vi "Inventory-Add#toIventory.vi"(7 "Quanity to Add/Subtract":i32, 8 "error in (no error)":errorcluster, 9 "Part Number In":string, 11 "ERP-Inventory in":refnum<class "ERP-Inventory.lvclass">) -> (0 "error out":errorcluster, 2 "Add-Converted to String":string, 3 "ERP-Inventory out":refnum<class "ERP-Inventory.lvclass">, 5 "Part Number Out":string)   [LabVIEW 2013, in "ERP-Inventory.lvclass"]
uses:
  ERP-Inventory.lvclass
  ERP-Inventory.lvclass/ERP-Inventory.ctl
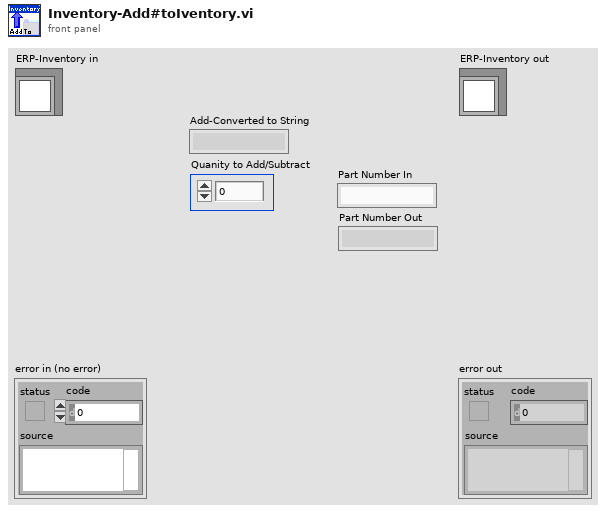
[diagram p1: front panel]
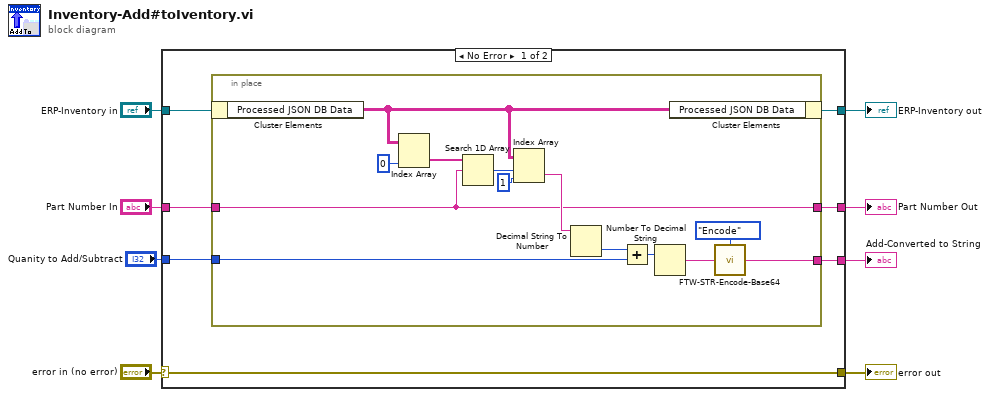
[diagram p0: block diagram]
diagram:
  n1 = case shown="No Error" "error in (no error)" {
    selector: "error in (no error)" -> [w15 w30]
    tunnel: [w15 w30] -> w7
    tunnel: [w12 w29] -> w5
    tunnel: "ERP-Inventory in" -> [w13 w29]
    tunnel: [w14 _] -> w4
    tunnel: "Quanity to Add/Subtract" -> [w11 _]
    tunnel: "Part Number In" -> [w10 _]
    tunnel: [w9 _] -> w1
    frame No Error {
      n2 = in-place {
        in-place-border: [w23] -> w14
        in-place-border: w11 -> [w27]
        in-place-border: w10 -> [w16]
        in-place-border: [w16] -> w9
        n3 = in-place-cluster #1(w13) -> ("Processed JSON DB Data"=w20:string[][])
        n4 = Index Array(array=w20, index (col)=0 ("disabled index (col)")) -> (element=w21:string[])  [unwired: 1 in]
        n5 = Search 1D Array(1D array=w21, element=w16) -> (index of element=w19:i32)  [unwired: 1 in]
        n6 = Index Array(array=w20, index (row)=w19, index (col)=1 ("disabled index (col)")) -> (element=w17:string)
        n7 = Decimal String To Number(string=w17) -> (number=w28:i32)  [unwired: 2 in, 1 out]
        n8 = Add(x=w28, y=w27) -> (x+y=w26:i32)
        n9 = Number To Decimal String(number=w26) -> (decimal integer string=w25:string)  [unwired: 1 in]
        n10 = in-place-cluster #1("Processed JSON DB Data"=w20) -> (w12:refnum<class "ERP-Inventory.lvclass">)
        n11 = call "FTW-STR-Encode-Base64.vi"("Input"=w25, "Direction"=enum16{"Encode", "Decode"}."Encode") -> ("Output"=w23:string)
      }
    }
    frame Error {
    }
  }
  "error out" <- w7
  "ERP-Inventory out" <- w5
  "Add-Converted to String" <- w4
  "Part Number Out" <- w1
